vi "LVFunction_Imop_SlopesPostProcessor_Apply NeighborExtension.vi"(0 "HasoSlopes in":refnum<class "HasoSlopes.lvclass">, 5 "HasoSlopes OUT":refnum<class "HasoSlopes.lvclass">, 11 "error in (no error)":errorcluster) -> (4 "HasoSlopes out":refnum<class "HasoSlopes.lvclass">, 6 "HasoSlopes OUT 2":refnum<class "HasoSlopes.lvclass">, 15 "error out":errorcluster)   [LabVIEW 2020]
doc: "Interpolates dark sub-pupils that are surrounded by light sub-pupils.\n\n<B>Slopes_inIn</B> : HasoSlopes object, modified by the processor if Slopes_out = NULL.\n<B>Slopes_inOut</B> : HasoSlopes object, modified by the processor if Slopes_out = NULL.\n<B>Slopes_out</B> : processed HasoSlopes object if not NULL."
uses:
  HasoSlopes.lvclass
  LVClass_HasoSlopes Read HasoSlopes _ property.vi
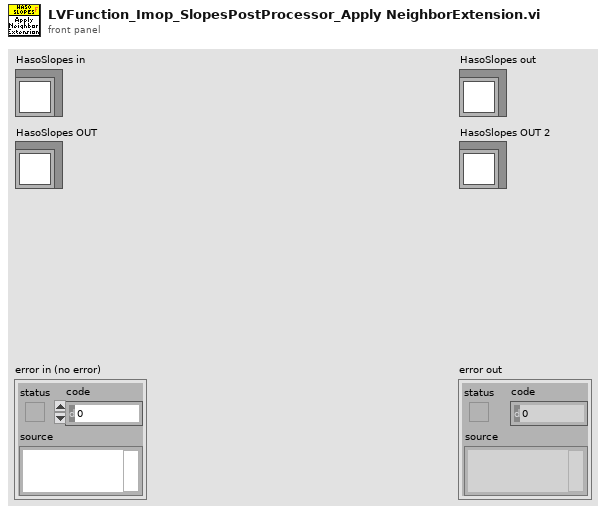
[diagram p1: front panel]
types:
  T1 = typedef "ClassID.ctl" = i64
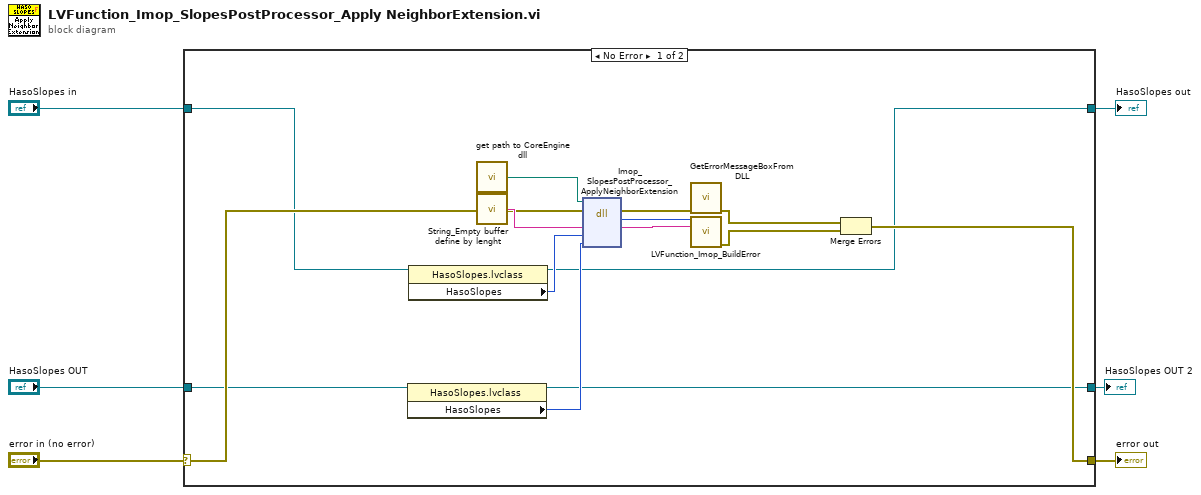
[diagram p0: block diagram]
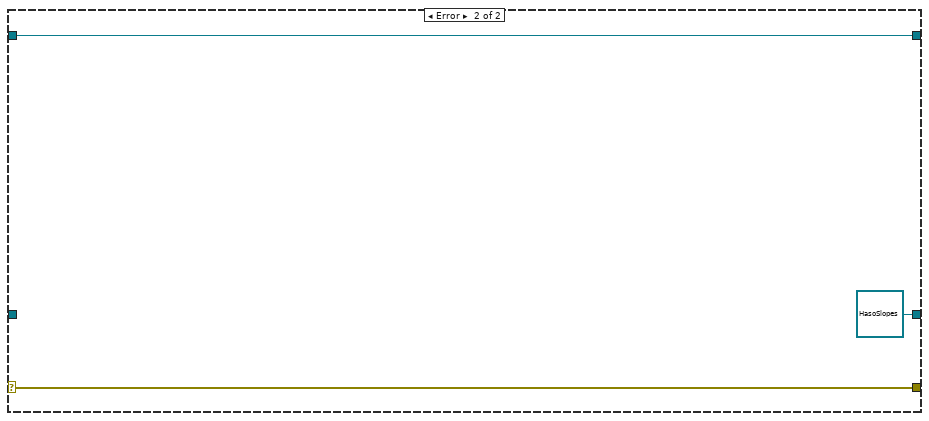
[diagram p2: hidden frame]
diagram:
  n1 = case shown="No Error" "error in (no error)" {
    selector: "error in (no error)" -> [w13 w24]
    tunnel: [w12 w24] -> w5
    tunnel: [w7 w23] -> w3
    tunnel: "HasoSlopes in" -> [w8 w23]
    tunnel: "HasoSlopes OUT" -> [w11 _]
    tunnel: [w9 refnum<class "HasoSlopes.lvclass"> refnum ("HasoSlopes OUT")] -> w1
    frame No Error {
      n2 = property class="HasoSlopes.lvclass"(reference=w11) -> (reference out=w9:refnum<class "HasoSlopes.lvclass">, "HasoSlopes"=w10:T1)  [unwired: 1 in, 1 out]
      n3 = property class="HasoSlopes.lvclass"(reference=w8) -> (reference out=w7:refnum<class "HasoSlopes.lvclass">, "HasoSlopes"=w21:T1)  [unwired: 1 in, 1 out]
      n4 = call "get path to CoreEngine dll.vi"() -> ("path to wavekit library"=w16:path)  [unwired: 14 in, 1 out]
      n5 = call "String_Empty buffer define by lenght.vi"() -> ("Empty buffer"=w17:string)  [unwired: 1 in]
      n6 = dll-call lib="D:/FLE/0.Code/CoreEngine4_Suite/LV2011_interface/DLLs/c_interface_vc100.dll" fn="Imop_SlopesPostProcessor_ApplyNeighborExtension"(path in=w16, error in=w13, "Message"=w17, "HasoSlopes IN"=w21, "HasoSlopes OUT"=w10) -> (error out=w20:errorcluster, "return type"=w18:i32, "Message"=w19:string)  [unwired: 3 in, 1 out]
      n7 = call "GetErrorMessageBoxFromDLL.vi"("error IN"=w20) -> ("error OUT"=w15:errorcluster)  [unwired: 10 in]
      n8 = call "LVFunction_Imop_BuildError.vi"("code"=w18, "String to Prepend to source (\"\")"=w19) -> ("error out"=w14:errorcluster)  [unwired: 13 in]
      n9 = Merge Errors(w15, w14) -> (w12:errorcluster)
    }
    frame Error {
    }
  }
  "error out" <- w5
  "HasoSlopes out" <- w3
  "HasoSlopes OUT 2" <- w1
